vi "Example Simple.vi"() -> ()   [LabVIEW 2010]
uses:
  C:/tf/play/labview/Tinkerforge.dll
panel:
  in  "uid":string="ioiu"
  in  "port":i32=4223
  in  "host":string="localhost"
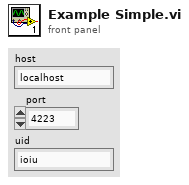
[diagram p1: front panel]
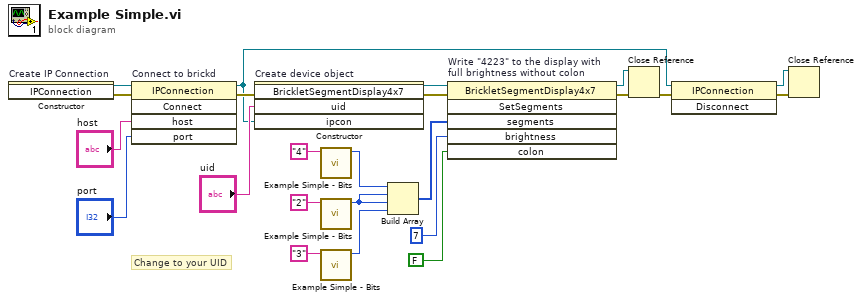
[diagram p0: block diagram]
diagram:
  # "Change to your UID"
  n1 = constructor on="Create IP Connection" class="IPConnection"() -> (reference out=w23:refnum<k24>, error out=w10:errorcluster)  [unwired: 3 in, 1 out]
  n2 = invoke on="Connect to brickd" class="IPConnection" method="Connect"(reference=w23, error in=w10, "host"="host", "port"="port") -> (reference out=w12:refnum<k24>, error out=w19:errorcluster)  [unwired: 1 in, 3 out]
  n3 = constructor on="Create device object" class="BrickletSegmentDisplay4x7"(error in=w19, "uid"="uid", "ipcon"=w12) -> (reference out=w17:refnum<k24>, error out=w18:errorcluster)  [unwired: 2 in, 3 out]
  n4 = call "Example Simple - Bits.vi"("character"="4") -> ("bits"=w6:u8)  [unwired: 10 in]
  n5 = call "Example Simple - Bits.vi"("character"="2") -> ("bits"=w3:u8)  [unwired: 10 in]
  n6 = call "Example Simple - Bits.vi"("character"="3") -> ("bits"=w1:u8)  [unwired: 10 in]
  n7 = Build Array(w6, w3, w3, w1) -> (w7:u8[])
  n8 = invoke on="Write \"4223\" to the display with\nfull brightness without colon" class="BrickletSegmentDisplay4x7" method="SetSegments"(reference=w17, error in=w18, "segments"=w7, "brightness"=u8 7, "colon"=FALSE) -> (reference out=w15:refnum<k24>, error out=w16:errorcluster)  [unwired: 1 in, 4 out]
  n9 = Close Reference(reference=w15, error in (no error)=w16) -> (error out=w14:errorcluster)
  n10 = invoke class="IPConnection" method="Disconnect"(reference=w12, error in=w14) -> (reference out=w11:refnum<k24>, error out=w13:errorcluster)  [unwired: 1 in, 1 out]
  n11 = Close Reference(reference=w11, error in (no error)=w13) -> ()  [unwired: 1 out]
